vi "DigitalTriggerApp.vi"() -> ()   [LabVIEW 2012]
uses:
  <vilib>/DAQmx/write.llb/DAQmx Write (Digital Bool 1Line 1Point).vi
  <vilib>/DAQmx/create/channels.llb/DAQmx Create Channel (DO-Digital Output).vi
  <vilib>/DAQmx/miscellaneous.llb/DAQmx Fill In Error Info.vi
  <vilib>/regexp/Match Regular Expression.xnode
panel:
  in  "Transparency":dbl(slide) scale=20.0..100.0
  out "LED":bool caption="OUTPUT"
  in  "TRIGGER":bool caption="TRG"
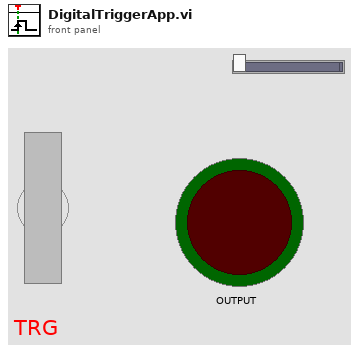
[diagram p1: front panel]
types:
  T1 = enum32{"invalid app kind", "Development System", "Run Time System", "Student Edition", "Embedded LabVIEW", "Evaluation", "Custom"}
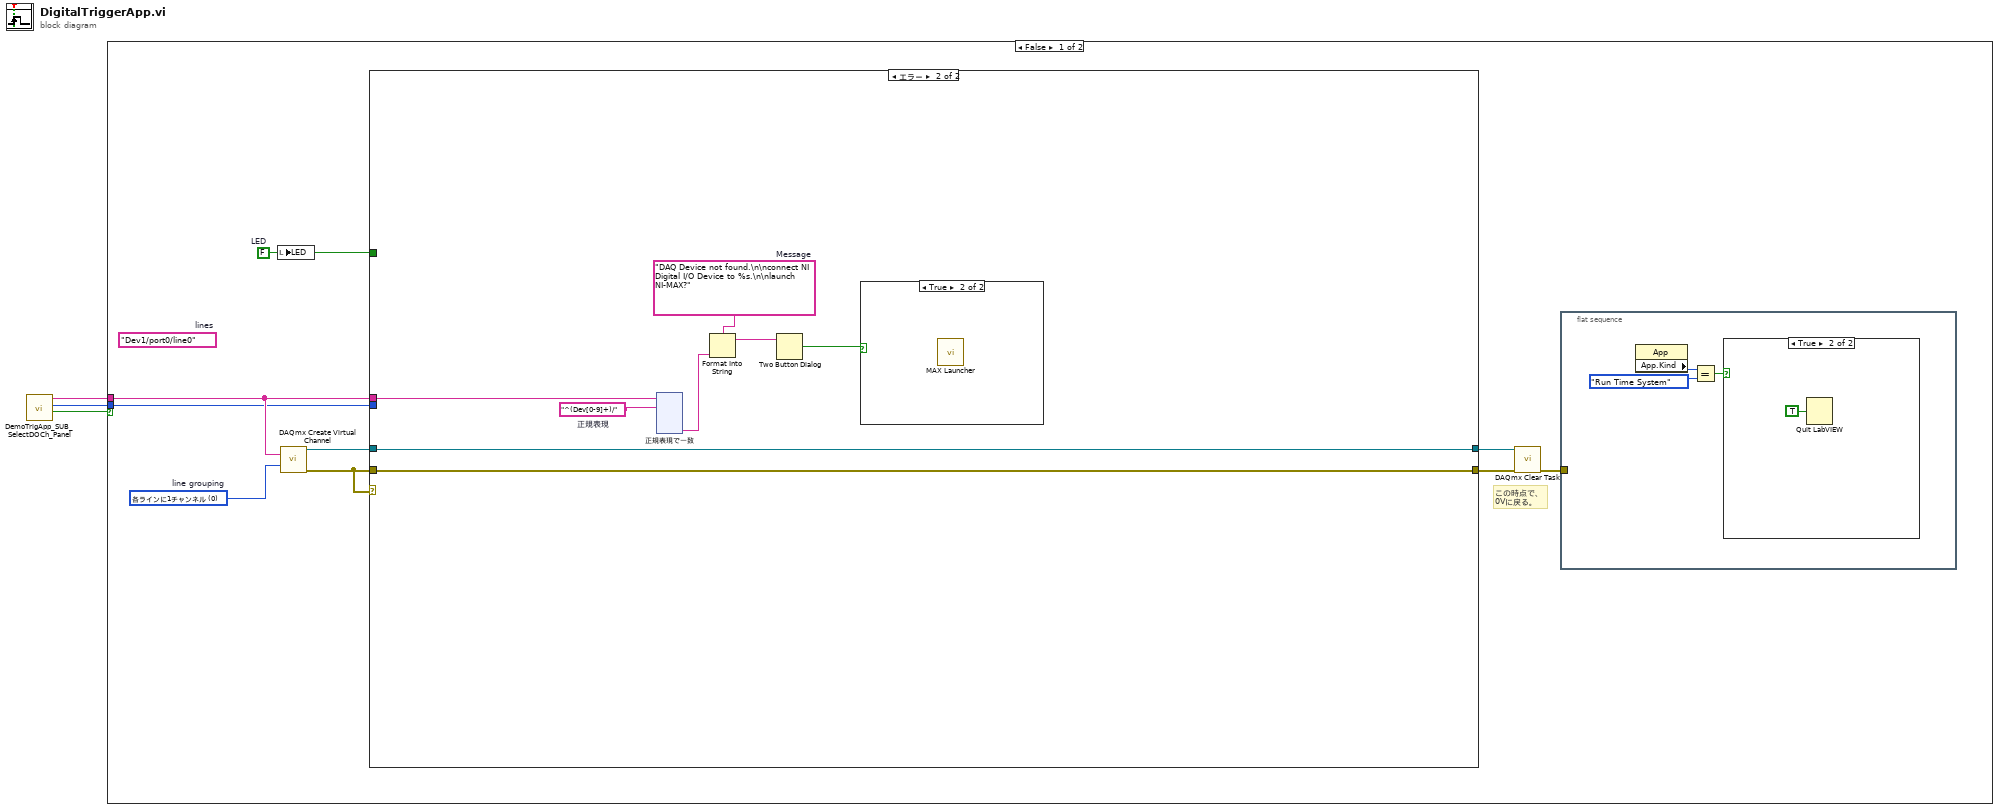
[diagram p0: block diagram]
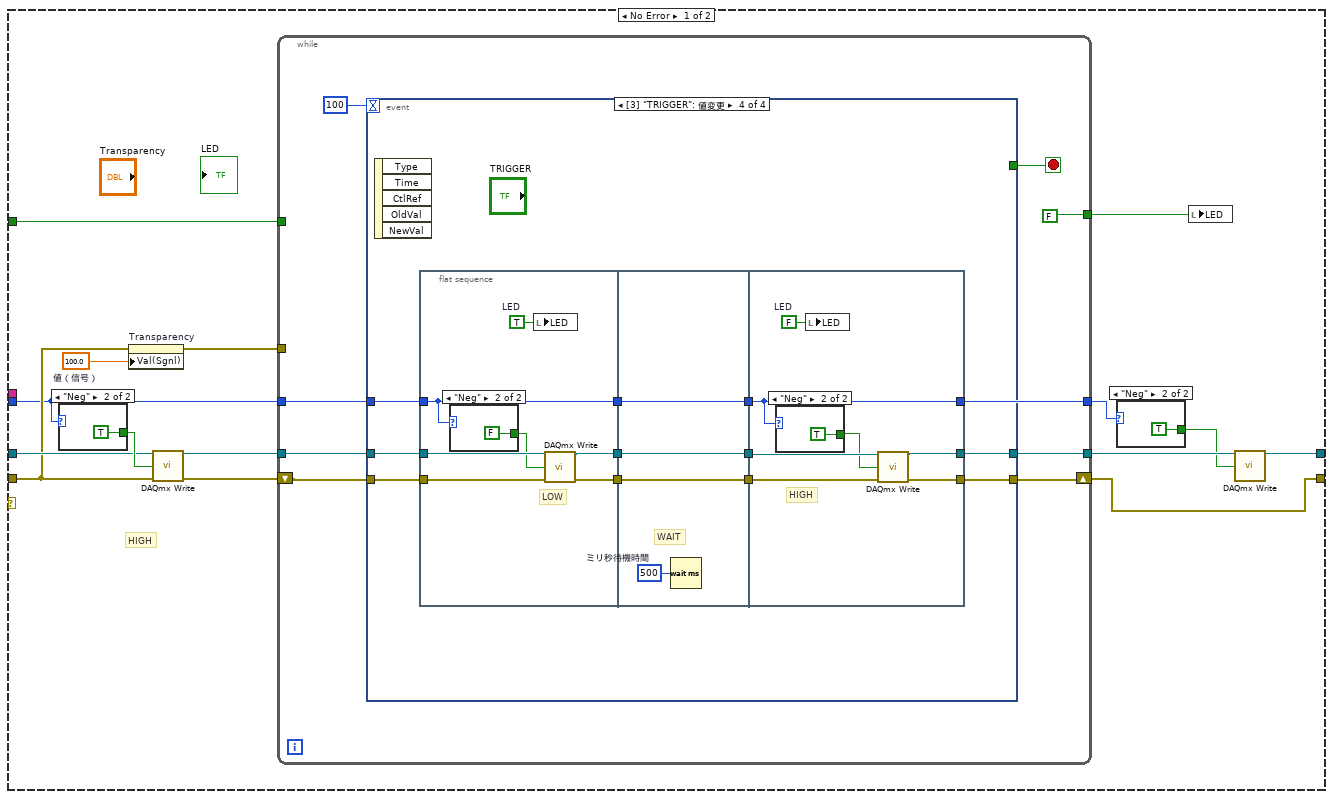
[diagram p3: hidden frame]
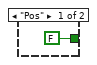
[diagram p4: hidden frame]
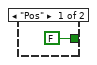
[diagram p5: hidden frame]
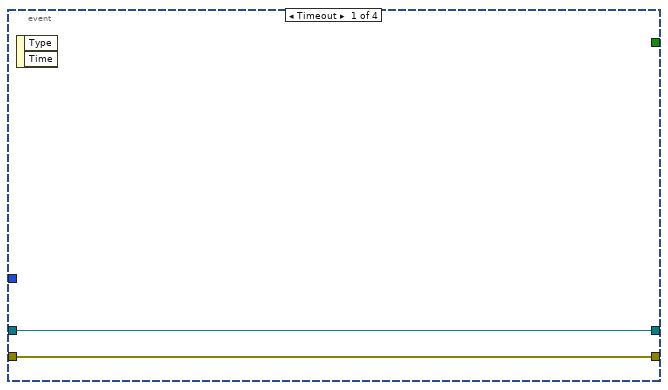
[diagram p6: hidden frame]
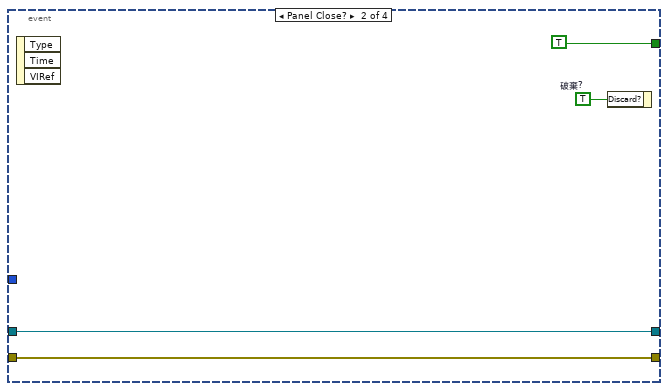
[diagram p7: hidden frame]
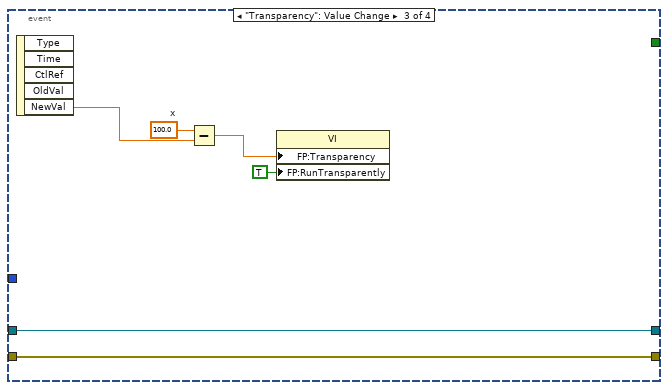
[diagram p8: hidden frame]
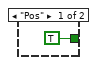
[diagram p9: hidden frame]
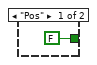
[diagram p10: hidden frame]
diagram:
  n1 = call "DemoTrigApp_SUB_SelectDOCh_Panel.vi"() -> ("Cancel"=w3:bool, "NegPos"=w1:enum16{"Neg", "Pos"}, "DO ch"=w2:tag)  [unwired: 9 in]
  n2 = case shown="FALSE" w3 {
    tunnel: w2 -> [w5 _]
    tunnel: w1 -> [w4 _]
    frame False {
      w10 = FALSE  # LED
      (unwired) tag "Dev1/port0/line0"  # lines
      w12 = 0 items=["各ラインに1チャンネル", "全てのラインに1チャンネル"]  # line grouping
      # "この時点で、\n0Vに戻る。"
      n3 = local write "LED"(w10) -> ()
      n4 = call-poly <vilib>:"DAQmx Create Virtual Channel.vi"("lines"=w5, "line grouping"=w12) -> ("task out"=w11:refnum<k21>, "error out"=w9:errorcluster)  [unwired: 12 in]
      n5 = case shown="エラー" w9 {
        tunnel: w11 -> [w25 w96]
        tunnel: w10 -> [w30 _]
        tunnel: w9 -> [w22 w95]
        tunnel: [w28 w96] -> w8
        tunnel: [w27 w95] -> w7
        tunnel: w5 -> [_ w93]
        tunnel: w4 -> [w19 _]
        frame No Error {
          w20 = 100.0  # 値（信号）
          # "HIGH"
          n6 = case shown="\"Neg\"" w19 {
            tunnel: [FALSE TRUE] -> w26
            frame "Pos" {
            }
            frame "Neg" {
            }
          }
          n7 = property on="Transparency" class="Slide （指定）"(error in=w22, "Val(Sgnl)"=w20) -> (error out=w21:errorcluster)  [unwired: 1 in, 1 out]
          n8 = call-poly <vilib>:"DAQmx Write.vi"("task/channels in"=w25, "data"=w26, "error in"=w22) -> ("task out"=w23:refnum<k21>, "error out"=w24:errorcluster)  [unwired: 10 in, 1 out]
          n9 = while {
            tunnel: [FALSE] -> w31
            tunnel: w23 -> [w40]
            tunnel: w30 -> [_]
            shift-right: [w38] -> w27
            shift-left: w24 -> [w39]
            tunnel: [w37] -> w29
            tunnel: w21 -> [_]
            tunnel: w19 -> [w36]
            tunnel: [w36] -> w17
            stop <- w42 stop-if-true
            n10 = event shown="[3] \"TRIGGER\": 値変更" {
              selector: _ -> [_ _ _ _]
              dyn-events: _ -> [_ _ _ _]
              timeout: 100 -> [_ _ _ _]
              tunnel: [_ TRUE _ _] -> w42
              tunnel: w40 -> [w44 w46 w54 w66]
              tunnel: w39 -> [w45 w47 w55 w65]
              tunnel: [w45 w47 w55 w64] -> w38
              tunnel: [w44 w46 w54 w61] -> w37
              tunnel: w36 -> [_ _ _ w58]
              event Timeout {
                n11 = event-data() -> ()  [unwired: 1 in, 2 out]
              }
              event Panel Close? {
                w49 = TRUE  # 破棄?
                n12 = event-data() -> ()  [unwired: 1 in, 3 out]
                n13 = event-data("Discard?"=w49) -> ()  [unwired: 1 in, 1 out]
              }
              event "Transparency": Value Change {
                w52 = 100.0  # x
                n14 = event-data() -> ("NewVal"=w51:dbl)  [unwired: 1 in, 4 out]
                n15 = Subtract(x=w52, y=w51) -> (x-y=w50:dbl)
                n16 = property class="VI"("FP:Transparency"=w50, "FP:RunTransparently"=TRUE) -> ()  [unwired: 2 in, 2 out]
              }
              event "TRIGGER": Value Change {
                n17 = event-data() -> ()  [unwired: 1 in, 5 out]
                n18 = flat-sequence {
                  tunnel: w66 -> [w72]
                  tunnel: w65 -> [w69]
                  tunnel: [w71] -> w60
                  tunnel: [w70] -> w59
                  tunnel: w58 -> [w68]
                  tunnel: [w68] -> w56
                  tunnel: [w78] -> w63
                  tunnel: [w77] -> w62
                  tunnel: w60 -> [w77]
                  tunnel: w59 -> [w78]
                  tunnel: [w76] -> w57
                  tunnel: w56 -> [w76]
                  tunnel: [w82] -> w64
                  tunnel: w63 -> [w84]
                  tunnel: [w83] -> w61
                  tunnel: w62 -> [w85]
                  tunnel: w57 -> [w81]
                  tunnel: [w81] -> _
                  frame #0 {
                    w73 = TRUE  # LED
                    # "LOW"
                    n19 = case shown="\"Neg\"" w68 {
                      tunnel: [TRUE FALSE] -> w67
                      frame "Pos" {
                      }
                      frame "Neg" {
                      }
                    }
                    n20 = local write "LED"(w73) -> ()
                    n21 = call-poly <vilib>:"DAQmx Write.vi"("task/channels in"=w72, "data"=w67, "error in"=w69) -> ("task out"=w71:refnum<k21>, "error out"=w70:errorcluster)  [unwired: 10 in, 1 out]
                  }
                  frame #1 {
                    w79 = u32 500  # ミリ秒待機時間
                    # "WAIT"
                    n22 = Wait (ms)(milliseconds to wait=w79) -> ()  [unwired: 1 out]
                  }
                  frame #2 {
                    w86 = FALSE  # LED
                    # "HIGH"
                    n23 = case shown="\"Neg\"" w81 {
                      tunnel: [FALSE TRUE] -> w80
                      frame "Pos" {
                      }
                      frame "Neg" {
                      }
                    }
                    n24 = local write "LED"(w86) -> ()
                    n25 = call-poly <vilib>:"DAQmx Write.vi"("task/channels in"=w85, "data"=w80, "error in"=w84) -> ("task out"=w83:refnum<k21>, "error out"=w82:errorcluster)  [unwired: 10 in, 1 out]
                  }
                }
              }
            }
          }
          n26 = case shown="\"Neg\"" w17 {
            tunnel: [FALSE TRUE] -> w18
            frame "Pos" {
            }
            frame "Neg" {
            }
          }
          n27 = local write "LED"(w31) -> ()
          n28 = call-poly <vilib>:"DAQmx Write.vi"("task/channels in"=w29, "data"=w18) -> ("task out"=w28:refnum<k21>)  [unwired: 11 in, 2 out]
        }
        frame Error {
          w94 = "^(Dev[0-9]+)/"  # 正規表現
          w92 = "DAQ Device not found.\n\nconnect NI Digital I/O Device to %s.\n\nlaunch NI-MAX?"  # Message
          n29 = xnode "正規表現で一致"("入力文字列"=w93, "正規表現"=w94) -> ("サブ一致 1"=w91:string)  [unwired: 4 in, 5 out]
          n30 = Format Into String(format string=w92, w91) -> (resulting string=w90:string)  [unwired: 2 in, 1 out]
          n31 = Two Button Dialog(message=w90) -> (T button?=w89:bool)  [unwired: 2 in]
          n32 = case shown="TRUE" w89 {
            frame False {
            }
            frame True {
              n33 = call "MAX Launcher.vi"() -> ()  [unwired: 1 in]
            }
          }
        }
      }
      n34 = call <vilib>:"DAQmx Clear Task.vi"("task in"=w8, "error in"=w7) -> ("error out"=w6:errorcluster)  [unwired: 13 in]
      n35 = flat-sequence {
        tunnel: w6 -> [_]
        frame #0 {
          n36 = property class="App"() -> ("App.Kind"=w15:T1)  [unwired: 2 in, 2 out]
          n37 = Equal?(x=w15, y=T1."Run Time System" ("アプリケーション:種類")) -> (x = y?=w13:bool)
          n38 = case shown="TRUE" w13 {
            frame False {
            }
            frame True {
              n39 = Quit LabVIEW(quit? (T)=TRUE ("終了?（T）")) -> ()
            }
          }
        }
      }
    }
    frame True {
    }
  }
